vi "aggregator - vii - complex - atomic.vi"(5 "aggregator action":T1, 7 "requested size":i32=20, 8 "number":cdb, 11 "state IN":T2={"requested size"=20, "Array"=[], "actual number of elements"=0}) -> (0 "slope":cdb, 1 "interp average":cdb, 2 "mean":cdb, 3 "state OUT":T2={"requested size"=20, "Array"=[], "actual number of elements"=0})   [LabVIEW 2018]
uses:
  interpolation state - real.ctl
  agregator -- action.ctl
  interpolation state - complex.ctl
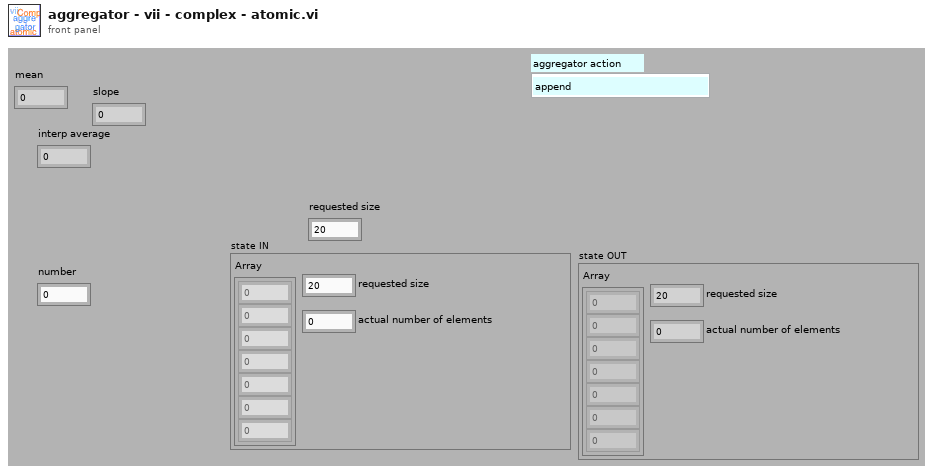
[diagram p1: front panel]
types:
  T1 = typedef "agregator -- action.ctl" = enum16{"append", "interpolate", "empty!", "force", "init", "scale", "read last"}
  T2 = typedef "interpolation state - complex.ctl" = cluster{"requested size":i32, "Array":cdb[], "actual number of elements":i32}
  T3 = typedef "interpolation state - real.ctl" = cluster{"requested size":i32, "Array":dbl[], "actual number of elements":i32}
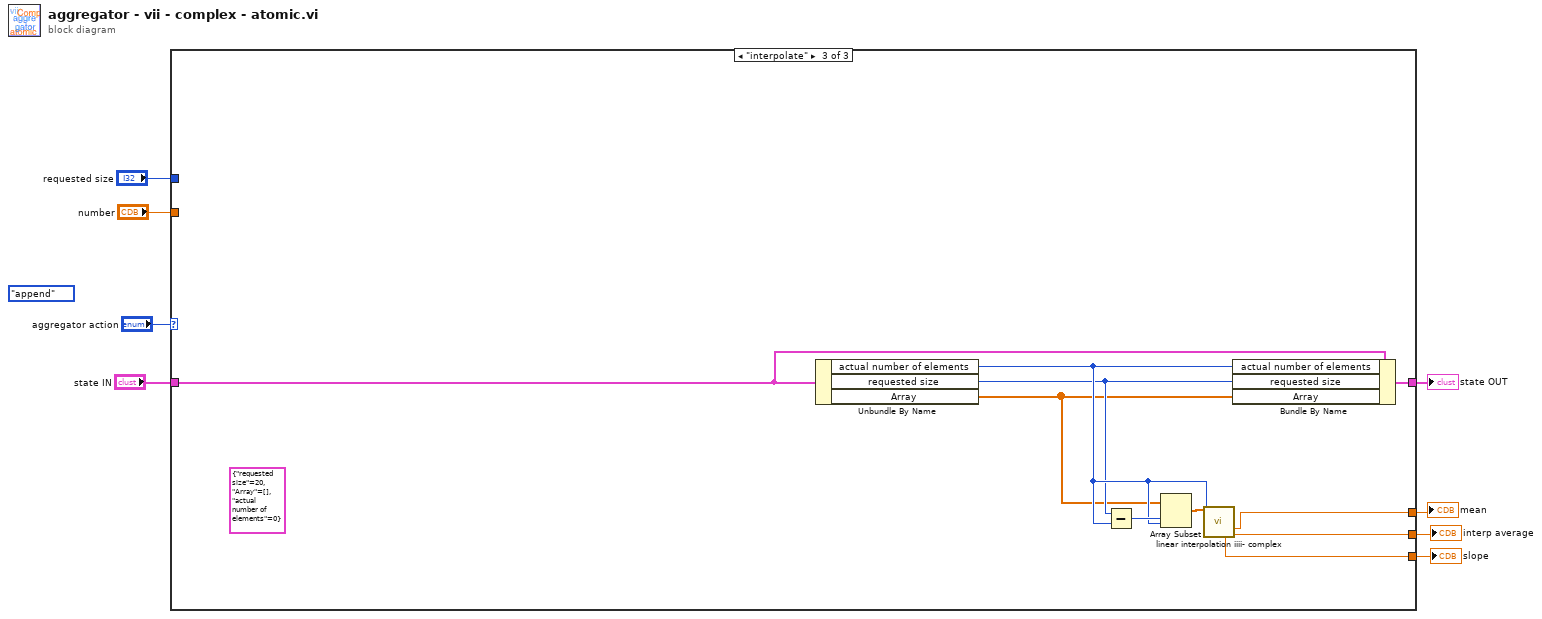
[diagram p0: block diagram]
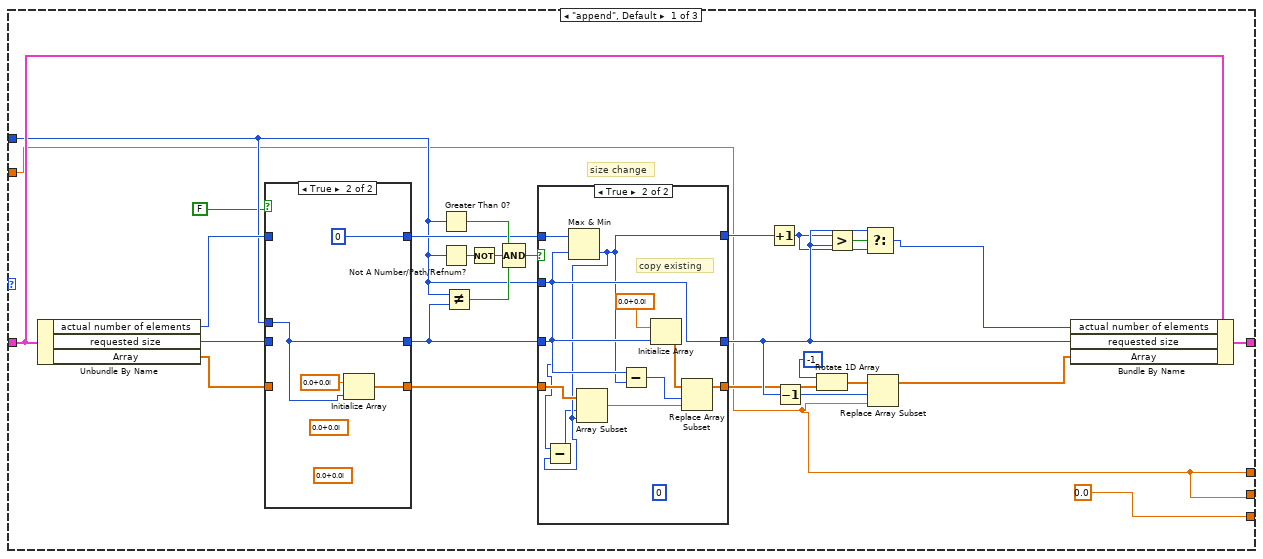
[diagram p2: hidden frame]
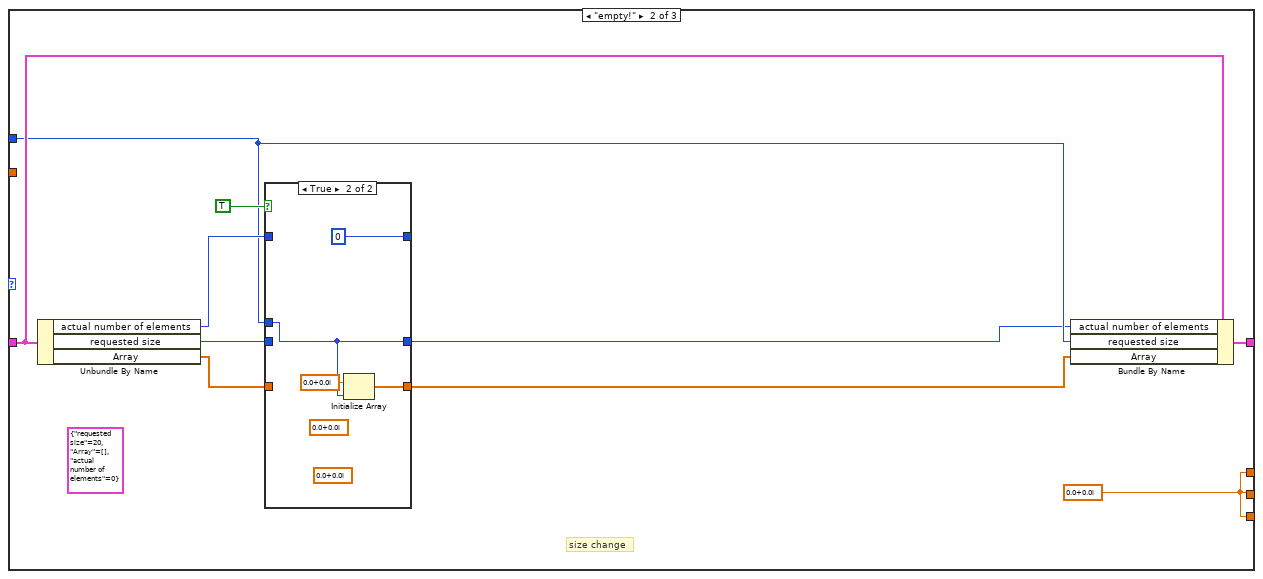
[diagram p5: hidden frame]
diagram:
  (unwired) agregator_--_action."append" ("aggregator action")
  n1 = case shown="\"interpolate\"" "aggregator action" {
    tunnel: [w9 w61 w83] -> w8
    tunnel: [w9 w61 w82] -> w7
    tunnel: [0.0 ("mean") w61 w81] -> w6
    tunnel: [w32 w63 w80] -> w5
    tunnel: "state IN" -> [w31 w62 w79]
    tunnel: "number" -> [w9 _ _]
    tunnel: "requested size" -> [w11 w58 _]
    frame "append", Default {
      # "size change"
      n2 = Unbundle By Name(w31) -> ("actual number of elements"=w34:i32, "requested size"=w35:i32, "Array"=w33:cdb[])
      n3 = case shown="True" FALSE {
        tunnel: w34 -> [w52 _]
        tunnel: [w52 0] -> w17
        tunnel: w33 -> [w50 _]
        tunnel: w11 -> [_ w53]
        tunnel: w35 -> [w51 _]
        tunnel: [w50 w54] -> w20
        tunnel: [w51 w53] -> w18
        frame False {
        }
        frame True {
          (unwired) cdb 0.0+0.0i
          (unwired) cdb 0.0+0.0i
          n4 = Initialize Array(cdb 0.0+0.0i, w53) -> (w54:cdb[])
        }
      }
      n5 = Greater Than 0?(x=w11) -> (x > 0?=w24:bool)
      n6 = Not A Number/Path/Refnum?(number/path/refnum=w11) -> (NaN/Path/Refnum?=w25:bool)
      n7 = Not Equal?(x=w11, y=w18) -> (x != y?=w22:bool)
      n8 = Not(x=w25) -> (.not. x?=w23:bool)
      n9 = Compound Arithmetic op=AND(w24, w23, w22) -> (w21:bool)
      n10 = case shown="True" w21 {
        tunnel: [w38 w40] -> w16
        tunnel: w17 -> [w38 w48]
        tunnel: [w37 w44] -> w29
        tunnel: w18 -> [w37 w41]
        tunnel: [w36 w47] -> w19
        tunnel: w20 -> [w36 w43]
        tunnel: w11 -> [_ w44]
        frame False {
        }
        frame True {
          (unwired) 0 ("disabled index (col)")
          # "copy existing"
          n11 = Max & Min(x=w48, y=w44) -> (min(x,y)=w40:i32)  [unwired: 1 out]
          n12 = Subtract(x=w41, y=w40) -> (x-y=w39:i32)
          n13 = Array Subset(array=w43, index=w39, length=w40) -> (w42:cdb[])
          n14 = Subtract(x=w44, y=w40) -> (x-y=w45:i32)
          n15 = Initialize Array(cdb 0.0+0.0i, w44) -> (w46:cdb[])
          n16 = Replace Array Subset(array=w46, new element=w42, index=w45) -> (w47:cdb[])
        }
      }
      n17 = Increment(x=w16) -> (x+1=w26:i32)
      n18 = Decrement(x=w29) -> (x-1=w14:i32)
      n19 = Rotate 1D Array(1:w19, 2:-1 ("n")) -> (0:w13:cdb[])
      n20 = Greater?(x=w26, y=w29) -> (0:w27:bool)
      n21 = Select(t=w29, s=w27, f=w26) -> (s? t:f=w30:i32)
      n22 = Replace Array Subset(array=w13, new element=w9, index=w14) -> (w28:cdb[])
      n23 = Bundle By Name(cluster=w31, "actual number of elements"=w30, "requested size"=w29, "Array"=w28) -> (w32:T2)
    }
    frame "empty!" {
      w61 = cdb 0.0+0.0i ("mean")
      (unwired) T3 {"requested size"=20, "Array"=[], "actual number of elements"=0} ("Cluster")
      # "size change"
      n24 = Unbundle By Name(w62) -> ("actual number of elements"=w65:i32, "requested size"=w66:i32, "Array"=w64:cdb[])
      n25 = case shown="True" TRUE {
        tunnel: w65 -> [w69 _]
        tunnel: [w69 0] -> _
        tunnel: w64 -> [w67 _]
        tunnel: w58 -> [_ w70]
        tunnel: w66 -> [w68 _]
        tunnel: [w67 w71] -> w59
        tunnel: [w68 w70] -> w57
        frame False {
        }
        frame True {
          (unwired) cdb 0.0+0.0i
          (unwired) cdb 0.0+0.0i
          n26 = Initialize Array(cdb 0.0+0.0i, w70) -> (w71:cdb[])
        }
      }
      n27 = Bundle By Name(cluster=w62, "actual number of elements"=w57, "requested size"=w58, "Array"=w59) -> (w63:T2)
    }
    frame "interpolate" {
      (unwired) T3 {"requested size"=20, "Array"=[], "actual number of elements"=0} ("Cluster")
      n28 = Unbundle By Name(w79) -> ("actual number of elements"=w76:i32, "requested size"=w75:i32, "Array"=w74:cdb[])
      n29 = Subtract(x=w75, y=w76) -> (x-y=w78:i32)
      n30 = Array Subset(array=w74, index=w78, length=w76) -> (w77:cdb[])
      n31 = call "linear interpolation iiii- complex.vi"("Array"=w77, "center"=w76) -> ("mean"=w83:cdb, "slope"=w81:cdb, "interpolated average"=w82:cdb)  [unwired: 5 in, 6 out]
      n32 = Bundle By Name(cluster=w79, "actual number of elements"=w76, "requested size"=w75, "Array"=w74) -> (w80:T2)
    }
  }
  "mean" <- w8
  "interp average" <- w7
  "slope" <- w6
  "state OUT" <- w5
